vi "FPGA_merFISH_trigger_camera_synchro_laser_lines_measure_QPD.vi"(3 "N Z positions":i32) -> ()   [LabVIEW 2015]
uses:
  <vilib>/Platform/TimedLoop/XDataNode/timing_clust.ctl
  <vilib>/Platform/TimedLoop/XDataNode/nitl_modes.ctl
  <vilib>/Platform/TimedLoop/XDataNode/wakeup.ctl
  <vilib>/rvi/FXPMathLib/basic elements/FxpIntAccumulator/subVIs/nifxpmath_IntAccumulator_SimConfig.ctl
  <vilib>/rvi/Emulation/niFpgaGetClockAttributes.vi
  <vilib>/rvi/Emulation/niFpgaSctlEmulationGetInTimedLoop.vi
  <vilib>/rvi/Emulation/niFpgaEmulationReportErrorSimple.vi
  <vilib>/rvi/eio/common/nirviEmuTemplateMethod_errors.vi
  <vilib>/rvi/Emulation/niFpgaProcessEmulError.vi
  <vilib>/rvi/Analysis/common/codeGenErrors/XNode/niFpgaXNodeCodeGenErrorHandle.vi
  <vilib>/rvi/Emulation/niFpgaCriticalErrorInLSC.vi
  <vilib>/rvi/FXPMathLib/basic elements/FxpIntAccumulator/simVIs/DllFxpIntAccumulator_sub.vi
  <vilib>/eio/EIONode/EIONode.xnode
  <vilib>/rvi/Analysis/measure/dc-rms/XNode/niFpgaDC-RMS.xnode
  <vilib>/Platform/TimedLoop/XDataNode/XDataNode.xnode
  <vilib>/rvi/FXPMathLib/basic elements/FxpIntAccumulator/XNode/nifxpmath_IntAccumulator.xnode
  <vilib>/Platform/TimedLoop/XDataNode/XDNodeRunTimeDep.lvlib
panel:
  out "n cycles":i32
  out "i":i32
  out "DIo1 2":i32
  out "DIo3":i32
  out "DIo1":i32
  in  "stop":bool
  out "duration (ms)":u32
  out "QPD":T1
  in  "Reset counter":bool
  out "Images acquired":i32
  in  "Laser lines":i32[](array[numeric])=[0, 0, 0, 0, 0]
  in  "Laser power":sgl[](array[numeric])=[0.0, 0.0, 0.0, 0.0, 0.0]
  in  "N laser lines":i32
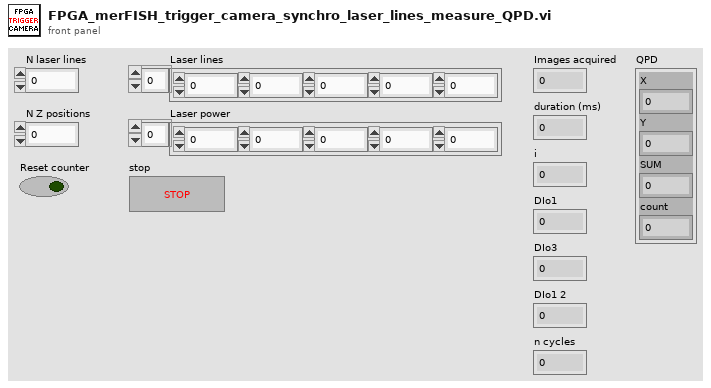
[diagram p1: front panel]
types:
  T1 = cluster{"X":sgl, "Y":sgl, "SUM":sgl, "count":u32}
  T2 = typedef "XDNodeRunTimeDep.lvlib/timing_clust.ctl" = cluster{"Expected End [f-1]":u64, "Actual End [f-1]":u64, "Finished Late? [f-1]":bool, "Expected End [i-1]":u64, "Actual End [i-1]":u64, "Finished Late? [i-1]":bool, "Expected Start [i]":u64, "Actual Start [i]":u64, "Expected Start [f]":u64, "Actual Start [f]":u64, "Source Name":string, "Structure Name":string, "Period":i64, "Deadline":i64, "Offset":i64, "Start":i64, "Priority":i32, "Timeout":i32, "Mode":T3, "Wakeup Reason":T4, "Error":errorcluster, "Source Type":string, "Secondary Source Type":string, "Global End Time":u64, "Global Start Time":u64, "Frame Duration":u64, "Iteration Duration":u64, "Assigned CPU":i32, "I/O Scan Engine Mode":u32}
  T3 = typedef "XDNodeRunTimeDep.lvlib/nitl_modes.ctl" = enum32{"No Change", "Process missed periods, maintain original phase", "Discard missed periods, maintain original phase", "Process missed periods, ignore original phase", "Discard missed periods, ignore original phase"}
  T4 = typedef "XDNodeRunTimeDep.lvlib/wakeup.ctl" = enum32{"Normal", "Aborted", "Asynchronous wakeup", "Timing source error", "Timed loop error", "Timeout"}
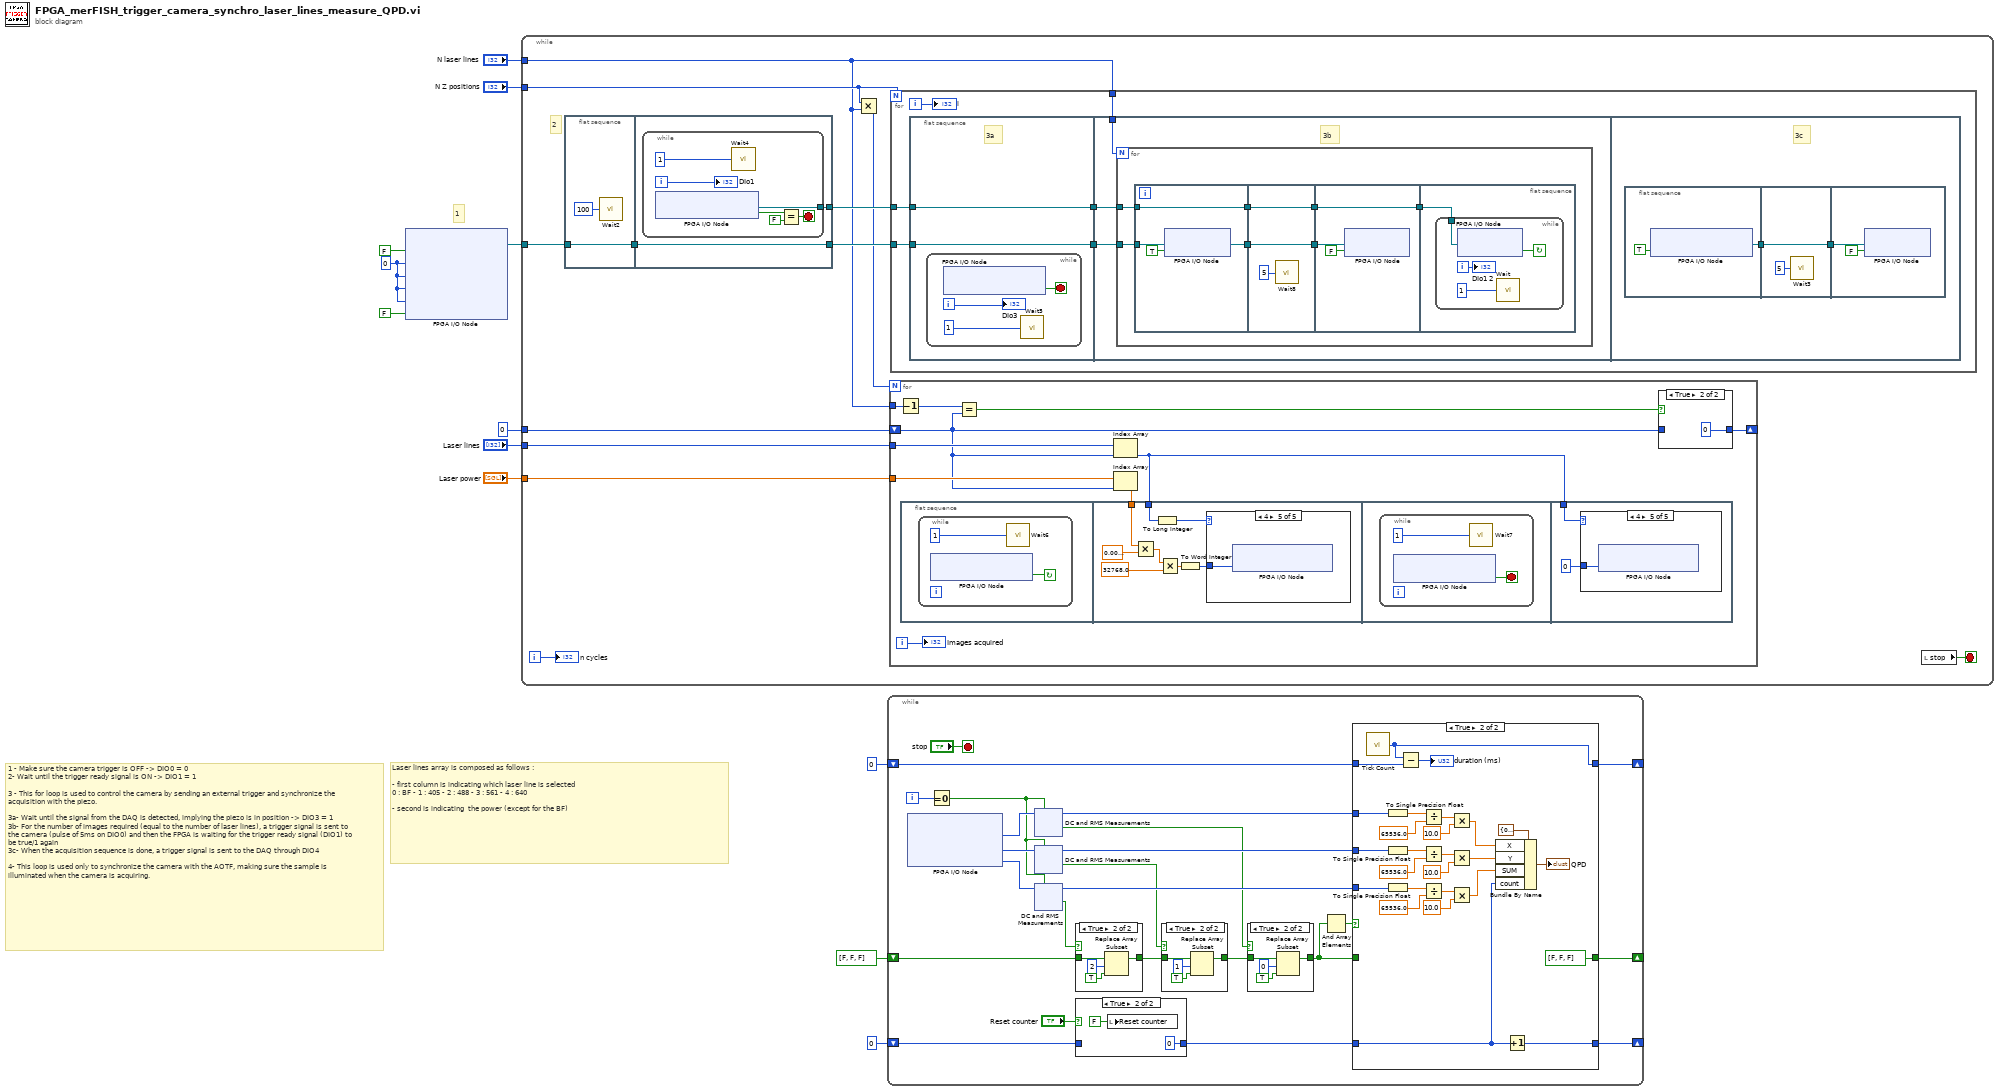
[diagram p0: block diagram]
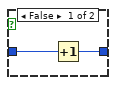
[diagram p2: hidden frame]
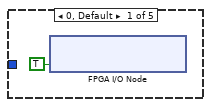
[diagram p3: hidden frame]
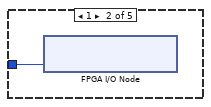
[diagram p4: hidden frame]
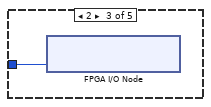
[diagram p5: hidden frame]
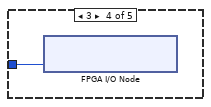
[diagram p6: hidden frame]
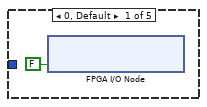
[diagram p7: hidden frame]
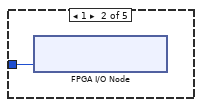
[diagram p8: hidden frame]
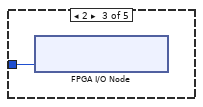
[diagram p9: hidden frame]
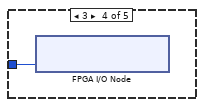
[diagram p10: hidden frame]
diagram:
  w5 = i16 0 ("Connector0/AO0")
  # "Laser lines array is composed as follows :\n\n- first column is indicating which laser line is selected \n0 : BF - 1 : 405 - 2 : 488 - 3 : 561 - 4 : 640\n\n- second is indicating  the power (except for the BF)"
  # "1"
  # "1 - Make sure the camera trigger is OFF -> DIO0 = 0\n2- Wait until the trigger ready signal is ON -> DIO1 = 1\n\n3 - This for loop is used to control the camera by sending an external trigger and synchronize the acquisition with the piezo.\n\n3a- Wait until the signal from the DAQ is detected, implying the piezo is in position -> DIO3 = 1 \n3b- For the number of images required (equal to the number of laser lines), a trigger signal is sent to the camera (pulse of 5ms on DIO0) and then the FPGA is waiting for the trigger ready signal (DIO1) to be true/1 again\n3c- When the acquisition sequence is done, a trigger signal is sent to the DAQ through DIO4\n\n4- This loop is used only to synchronize the camera with the AOTF, making sure the sample is illuminated when the camera is acquiring."
  n1 = xnode "FPGA I/O Node"("Connector0/DIO0"=FALSE, "Connector0/AO0"=w5, "Connector0/AO1"=w5, "Connector0/AO2"=w5, "Connector0/AO3"=w5, "Connector0/DIO5"=FALSE) -> ("FPGA I/O Out"=w11:refnum<k21>)  [unwired: 6 in, 5 out]
  n2 = while {
    tunnel: w11 -> [w23]
    tunnel: "Laser power" -> [w20]
    tunnel: "Laser lines" -> [w19]
    tunnel: 0 -> [w18]
    tunnel: "N Z positions" -> [w17]
    tunnel: "N laser lines" -> [w15]
    i -> [w13]
    stop <- w14 stop-if-true
    # "2"
    n3 = flat-sequence {
      tunnel: w23 -> [w63]
      tunnel: [w63] -> w24
      tunnel: w24 -> [w65]
      tunnel: [w65] -> w22
      tunnel: [w64] -> w21
      frame #0 {
        n4 = call "Wait2"("Count(uSec)"=u32 100 ("Count(mSec)")) -> ()  [unwired: 1 out]
      }
      frame #1 {
        n5 = while {
          tunnel: [w71] -> w64
          i -> [w67]
          stop <- w68 stop-if-true
          n6 = xnode "FPGA I/O Node"() -> ("Connector0/DIO1"=w70:bool, "FPGA I/O Out"=w71:refnum<k21>)  [unwired: 1 in]
          n7 = call "Wait4"("Count(mSec)"=u32 1) -> ()  [unwired: 1 out]
          n8 = Equal?(x=w70, y=FALSE) -> (x = y?=w68:bool)
          "DIo1" <- w67
        }
      }
    }
    n9 = Multiply(x=w17, y=w15) -> (x*y=w16:i32)
    n10 = for {
      N: w16 -> [_]
      shift-right: [w32] -> _
      shift-left: w18 -> [w29]
      tunnel: w19 -> [w31]
      tunnel: w20 -> [w30]
      tunnel: w15 -> [w27]
      i -> [w25]
      n11 = Decrement(x=w27) -> (x-1=w26:i32)
      n12 = flat-sequence {
        tunnel: w34 -> [w42]
        tunnel: w28 -> [w41]
        tunnel: w34 -> [w55]
        frame #0 {
          n13 = while {
            stop <- w39 continue-if-true
            n14 = xnode "FPGA I/O Node"() -> ("Connector0/DIO2"=w39:bool)  [unwired: 1 in, 1 out]
            n15 = call "Wait6"("Count(mSec)"=u32 1) -> ()  [unwired: 1 out]
          }
        }
        frame #1 {
          n16 = Multiply(x=w41, y=sgl 0.01) -> (x*y=w40:sgl)
          n17 = To Long Integer(number=w42) -> (32bit integer=w47:i32)
          n18 = Multiply(x=w40, y=sgl 32768.0) -> (x*y=w44:sgl)
          n19 = To Word Integer(number=w44) -> (16bit integer=w43:i16)
          n20 = case shown="4" w47 {
            tunnel: w43 -> [_ w49 w50 w51 w52]
            frame 0, Default {
              n21 = xnode "FPGA I/O Node"("Connector0/DIO5"=TRUE) -> ()  [unwired: 1 in, 1 out]
            }
            frame 1 {
              n22 = xnode "FPGA I/O Node"("Connector0/AO2"=w49) -> ()  [unwired: 1 in, 1 out]
            }
            frame 2 {
              n23 = xnode "FPGA I/O Node"("Connector0/AO3"=w50) -> ()  [unwired: 1 in, 1 out]
            }
            frame 3 {
              n24 = xnode "FPGA I/O Node"("Connector0/AO0"=w51) -> ()  [unwired: 1 in, 1 out]
            }
            frame 4 {
              n25 = xnode "FPGA I/O Node"("Connector0/AO1"=w52) -> ()  [unwired: 1 in, 1 out]
            }
          }
        }
        frame #2 {
          n26 = while {
            stop <- w54 stop-if-true
            n27 = xnode "FPGA I/O Node"() -> ("Connector0/DIO2"=w54:bool)  [unwired: 1 in, 1 out]
            n28 = call "Wait7"("Count(mSec)"=u32 1) -> ()  [unwired: 1 out]
          }
        }
        frame #3 {
          n29 = case shown="4" w55 {
            tunnel: i16 0 -> [_ w58 w59 w60 w61]
            frame 0, Default {
              n30 = xnode "FPGA I/O Node"("Connector0/DIO5"=FALSE) -> ()  [unwired: 1 in, 1 out]
            }
            frame 1 {
              n31 = xnode "FPGA I/O Node"("Connector0/AO2"=w58) -> ()  [unwired: 1 in, 1 out]
            }
            frame 2 {
              n32 = xnode "FPGA I/O Node"("Connector0/AO3"=w59) -> ()  [unwired: 1 in, 1 out]
            }
            frame 3 {
              n33 = xnode "FPGA I/O Node"("Connector0/AO0"=w60) -> ()  [unwired: 1 in, 1 out]
            }
            frame 4 {
              n34 = xnode "FPGA I/O Node"("Connector0/AO1"=w61) -> ()  [unwired: 1 in, 1 out]
            }
          }
        }
      }
      n35 = Equal?(x=w26, y=w29) -> (x = y?=w33:bool)
      n36 = Index Array(array=w31, index=w29) -> (element=w34:i32)
      n37 = Index Array(array=w30, index=w29) -> (element=w28:sgl)
      n38 = case shown="True" w33 {
        tunnel: w29 -> [w36 _]
        tunnel: [w35 0] -> w32
        frame False {
          n39 = Increment(x=w36) -> (x+1=w35:i32)
        }
        frame True {
        }
      }
      "Images acquired" <- w25
    }
    n40 = for {
      N: w17 -> [_]
      tunnel: w22 -> [w76]
      tunnel: w21 -> [w77]
      tunnel: w15 -> [w73]
      i -> [w72]
      n41 = flat-sequence {
        tunnel: w76 -> [w78]
        tunnel: w77 -> [w79]
        tunnel: [w79] -> w75
        tunnel: [w78] -> w74
        tunnel: w75 -> [w85]
        tunnel: w74 -> [w84]
        tunnel: w73 -> [w83]
        frame #0 {
          # "3a"
          n42 = while {
            i -> [w81]
            stop <- w82 stop-if-true
            n43 = xnode "FPGA I/O Node"() -> ("Connector0/DIO3"=w82:bool)  [unwired: 1 in, 1 out]
            n44 = call "Wait5"("Count(mSec)"=u32 1) -> ()  [unwired: 1 out]
            "DIo3" <- w81
          }
        }
        frame #1 {
          # "3b"
          n45 = for {
            N: w83 -> [_]
            tunnel: w85 -> [w87]
            tunnel: w84 -> [w86]
            n46 = flat-sequence {
              tunnel: [w95] -> w92
              tunnel: [w93] -> w91
              tunnel: w86 -> [w94]
              tunnel: w87 -> [w93]
              tunnel: w92 -> [w99]
              tunnel: [w99] -> w90
              tunnel: [w98] -> w89
              tunnel: w91 -> [w98]
              tunnel: w90 -> [w101]
              tunnel: [w100] -> w88
              tunnel: w89 -> [w100]
              tunnel: w88 -> [w103]
              frame #0 {
                n47 = xnode "FPGA I/O Node"("I/O Item"=TRUE ("Connector0/DIO0"), "FPGA I/O In"=w94) -> ("FPGA I/O Out"=w95:refnum<k21>)
              }
              frame #1 {
                n48 = call "Wait8"("Count(mSec)"=u32 5) -> ()  [unwired: 1 out]
              }
              frame #2 {
                n49 = xnode "FPGA I/O Node"("I/O Item"=FALSE ("Connector0/DIO0"), "FPGA I/O In"=w101) -> ()  [unwired: 1 out]
              }
              frame #3 {
                n50 = while {
                  tunnel: w103 -> [w107]
                  i -> [w105]
                  stop <- w106 continue-if-true
                  n51 = xnode "FPGA I/O Node"("FPGA I/O In"=w107) -> ("I/O Item"=w106:bool)  [unwired: 1 out]
                  n52 = call "Wait"("Count(mSec)"=u32 1) -> ()  [unwired: 1 out]
                  "DIo1 2" <- w105
                }
              }
            }
          }
        }
        frame #2 {
          # "3c"
          n53 = flat-sequence {
            tunnel: [w111] -> w109
            tunnel: w109 -> [w112]
            tunnel: [w112] -> w108
            tunnel: w108 -> [w114]
            frame #0 {
              n54 = xnode "FPGA I/O Node"("Connector0/DIO4"=TRUE) -> ("FPGA I/O Out"=w111:refnum<k21>)  [unwired: 1 in]
            }
            frame #1 {
              n55 = call "Wait3"("Count(mSec)"=u32 5) -> ()  [unwired: 1 out]
            }
            frame #2 {
              n56 = xnode "FPGA I/O Node"("I/O Item"=FALSE ("Connector0/DIO0"), "FPGA I/O In"=w114) -> ()  [unwired: 1 out]
            }
          }
        }
      }
      "i" <- w72
    }
    n57 = local read "stop"() -> (w14:bool)
    "n cycles" <- w13
  }
  n58 = while {
    shift-right: [w122] -> _
    shift-left: bool[] [FALSE, FALSE, FALSE] ("initialized array") -> [w130]
    shift-right: [w120] -> _
    shift-left: u32 0 -> [w121]
    shift-right: [w119] -> _
    shift-left: u32 0 -> [w117]
    i -> [w137]
    stop <- "stop" stop-if-true
    n59 = xnode "FPGA I/O Node"() -> ("Connector0/AI0"=w139:i16, "Connector0/AI1"=w135:i16, "Connector0/AI2"=w134:i16)  [unwired: 3 in, 3 out]
    n60 = Equal To 0?(x=w137) -> (x = 0?=w131:bool)
    n61 = xnode "DC and RMS Measurements"("input data"=w139, "reset"=w131) -> ("DC"=w136:i16, "output valid"=w125:bool)
    n62 = xnode "DC and RMS Measurements"("input data"=w135, "reset"=w131) -> ("DC"=w133:i16, "output valid"=w126:bool)
    n63 = xnode "DC and RMS Measurements"("input data"=w134, "reset"=w131) -> ("DC"=w132:i16, "output valid"=w127:bool)
    n64 = case shown="True" w127 {
      tunnel: w130 -> [w148 w151]
      tunnel: [w148 w149] -> w129
      frame False {
      }
      frame True {
        n65 = Replace Array Subset(array=w151, new element=TRUE, index=2) -> (w149:bool[])
      }
    }
    n66 = case shown="True" "Reset counter" {
      tunnel: w117 -> [w140 _]
      tunnel: [w140 u32 0] -> w116
      frame False {
      }
      frame True {
        n67 = local write "Reset counter"(FALSE ("Reset counter")) -> ()
      }
    }
    n68 = case shown="True" w126 {
      tunnel: w129 -> [w153 w156]
      tunnel: [w153 w154] -> w128
      frame False {
      }
      frame True {
        n69 = Replace Array Subset(array=w156, new element=TRUE, index=1) -> (w154:bool[])
      }
    }
    n70 = case shown="True" w125 {
      tunnel: [w143 w145] -> w123
      tunnel: w128 -> [w143 w144]
      frame False {
      }
      frame True {
        n71 = Replace Array Subset(array=w144, new element=TRUE, index=0) -> (w145:bool[])
      }
    }
    n72 = And Array Elements(Boolean array=w123) -> (logical AND=w124:bool)
    n73 = case shown="True" w124 {
      tunnel: w136 -> [_ w186]
      tunnel: w133 -> [_ w177]
      tunnel: w132 -> [_ w172]
      tunnel: w123 -> [w160 _]
      tunnel: [w160 bool[] [FALSE, FALSE, FALSE] ("initialized array")] -> w122
      tunnel: w121 -> [w159 w167]
      tunnel: [w159 w165] -> w120
      tunnel: w116 -> [w158 w162]
      tunnel: [w158 w161] -> w119
      frame False {
      }
      frame True {
        n74 = call "Tick Count"() -> ("Tick Count(mSec)"=w165:u32)
        n75 = To Single Precision Float(number=w186) -> (single precision float=w185:sgl)
        n76 = To Single Precision Float(number=w177) -> (single precision float=w178:sgl)
        n77 = To Single Precision Float(number=w172) -> (single precision float=w176:sgl)
        n78 = Subtract(x=w165, y=w167) -> (x-y=→"duration (ms)":u32)
        n79 = Divide(x=w185, y=sgl 65536.0) -> (x/y=w183:sgl)
        n80 = Divide(x=w178, y=sgl 65536.0) -> (x/y=w180:sgl)
        n81 = Divide(x=w176, y=sgl 65536.0) -> (x/y=w174:sgl)
        n82 = Multiply(x=w183, y=sgl 10.0) -> (x*y=w171:sgl)
        n83 = Multiply(x=w180, y=sgl 10.0) -> (x*y=w170:sgl)
        n84 = Multiply(x=w174, y=sgl 10.0) -> (x*y=w169:sgl)
        n85 = Bundle By Name(cluster=T1 {"X"=0.0, "Y"=0.0, "SUM"=0.0, "count"=0} ("output cluster"), "X"=w171, "Y"=w170, "SUM"=w169, "count"=w162) -> (→"QPD":T1)
        n86 = Increment(x=w162) -> (x+1=w161:u32)
      }
    }
  }
